vi "FormatHexValue.vi"(10 "Value":i16) -> (2 "FormattedValue":string)   [LabVIEW 2017, in "Thermal Shock.lvlib"]
uses:
  Thermal Shock.lvlib
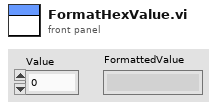
[diagram p1: front panel]
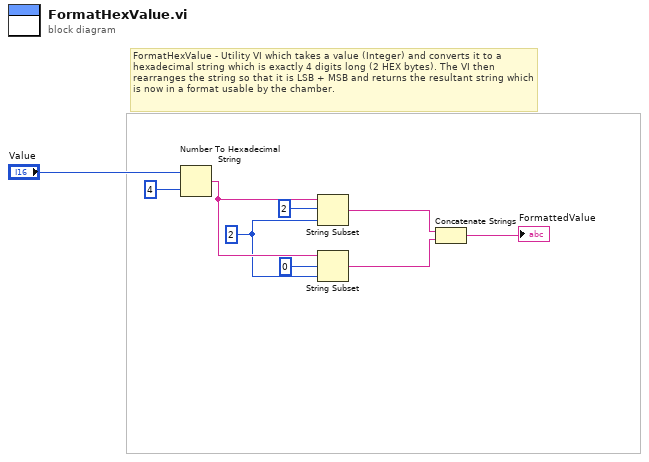
[diagram p0: block diagram]
diagram:
  w6 = 2
  # "FormatHexValue - Utility VI which takes a value (Integer) and converts it to a hexadecimal string which is exactly 4 digits long (2 HEX bytes). The VI then rearranges the string so that it is LSB + MSB and returns the resultant string which is now in a format usable by the chamber."
  n1 = Number To Hexadecimal String(1:4, 2:"Value") -> (0:w7:string)
  n2 = String Subset(string=w7, offset (0)=2, length (rest)=w6) -> (substring=w3:string)
  n3 = String Subset(string=w7, offset (0)=0, length (rest)=w6) -> (substring=w2:string)
  n4 = Concatenate Strings(w3, w2) -> (→"FormattedValue":string)
